vi "Update Position.vi"(10 "Direction":T2, 11 "Position in":T1) -> (3 "Position out":T1)   [LabVIEW 2015, in "Common.lvlib"]
uses:
  Common.lvlib
  Position.ctl
  Type Defs/Direction Enum.ctl
  SubVIs/Read-Only Globals.vi
  SubVIs/Globals (private).vi
  Square/Square.lvclass
  Type Defs/SB Type Defs.lvlib
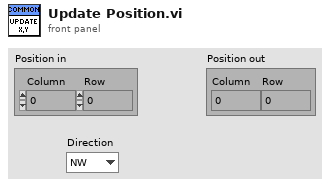
[diagram p1: front panel]
types:
  T1 = typedef "Common.lvlib/Position.ctl" = cluster{"Column":i32, "Row":i32}
  T2 = typedef "SB Type Defs.lvlib/Direction Enum.ctl" = enum16{"NW", "N", "NE", "E", "SE", "S", "SW", "W"}
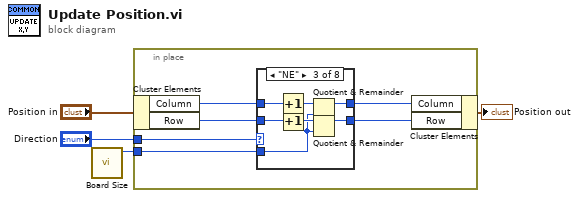
[diagram p0: block diagram]
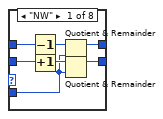
[diagram p2: hidden frame]
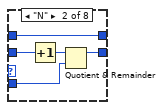
[diagram p3: hidden frame]
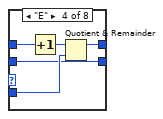
[diagram p4: hidden frame]
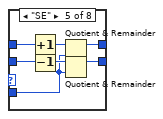
[diagram p5: hidden frame]
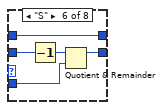
[diagram p6: hidden frame]
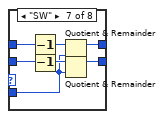
[diagram p7: hidden frame]
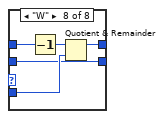
[diagram p8: hidden frame]
diagram:
  n1 = call "Board Size.vi"() -> ("Board Size"=w3:i32)  [unwired: 11 in]
  n2 = in-place {
    in-place-border: "Direction" -> [w10]
    in-place-border: w3 -> [w7]
    n3 = in-place-cluster #1("Position in") -> ("Column"=w9:i32, "Row"=w8:i32)
    n4 = case shown="\"NE\"" w10 {
      tunnel: w9 -> [w16 w18 w28 w34 w40 w42 w52 w58]
      tunnel: w8 -> [w17 w22 w29 w30 w41 w46 w53 w54]
      tunnel: [w14 w20 w26 w30 w38 w44 w50 w54] -> w6
      tunnel: [w11 w18 w23 w31 w35 w42 w47 w55] -> w5
      tunnel: w7 -> [w12 w19 w24 w32 w36 w43 w48 w56]
      frame "NW" {
        n5 = Decrement(x=w16) -> (x-1=w13:i32)
        n6 = Increment(x=w17) -> (x+1=w15:i32)
        n7 = Quotient & Remainder(x=w13, y=w12) -> (x-y*floor(x/y)=w11:i32)  [unwired: 1 out]
        n8 = Quotient & Remainder(x=w15, y=w12) -> (x-y*floor(x/y)=w14:i32)  [unwired: 1 out]
      }
      frame "N" {
        n9 = Increment(x=w22) -> (x+1=w21:i32)
        n10 = Quotient & Remainder(x=w21, y=w19) -> (x-y*floor(x/y)=w20:i32)  [unwired: 1 out]
      }
      frame "NE" {
        n11 = Increment(x=w28) -> (x+1=w25:i32)
        n12 = Increment(x=w29) -> (x+1=w27:i32)
        n13 = Quotient & Remainder(x=w25, y=w24) -> (x-y*floor(x/y)=w23:i32)  [unwired: 1 out]
        n14 = Quotient & Remainder(x=w27, y=w24) -> (x-y*floor(x/y)=w26:i32)  [unwired: 1 out]
      }
      frame "E" {
        n15 = Increment(x=w34) -> (x+1=w33:i32)
        n16 = Quotient & Remainder(x=w33, y=w32) -> (x-y*floor(x/y)=w31:i32)  [unwired: 1 out]
      }
      frame "SE" {
        n17 = Increment(x=w40) -> (x+1=w37:i32)
        n18 = Decrement(x=w41) -> (x-1=w39:i32)
        n19 = Quotient & Remainder(x=w37, y=w36) -> (x-y*floor(x/y)=w35:i32)  [unwired: 1 out]
        n20 = Quotient & Remainder(x=w39, y=w36) -> (x-y*floor(x/y)=w38:i32)  [unwired: 1 out]
      }
      frame "S" {
        n21 = Decrement(x=w46) -> (x-1=w45:i32)
        n22 = Quotient & Remainder(x=w45, y=w43) -> (x-y*floor(x/y)=w44:i32)  [unwired: 1 out]
      }
      frame "SW" {
        n23 = Decrement(x=w52) -> (x-1=w49:i32)
        n24 = Decrement(x=w53) -> (x-1=w51:i32)
        n25 = Quotient & Remainder(x=w49, y=w48) -> (x-y*floor(x/y)=w47:i32)  [unwired: 1 out]
        n26 = Quotient & Remainder(x=w51, y=w48) -> (x-y*floor(x/y)=w50:i32)  [unwired: 1 out]
      }
      frame "W" {
        n27 = Decrement(x=w58) -> (x-1=w57:i32)
        n28 = Quotient & Remainder(x=w57, y=w56) -> (x-y*floor(x/y)=w55:i32)  [unwired: 1 out]
      }
    }
    n29 = in-place-cluster #1("Column"=w5, "Row"=w6) -> (→"Position out":T1)
  }
